vi "Binary.vi"(8 "Angle":dbl, 11 "General settings":T1) -> (2 "Binary":dbl[][](array[numeric]))   [LabVIEW 2014]
uses:
  Controls/SLM General Settings.ctl
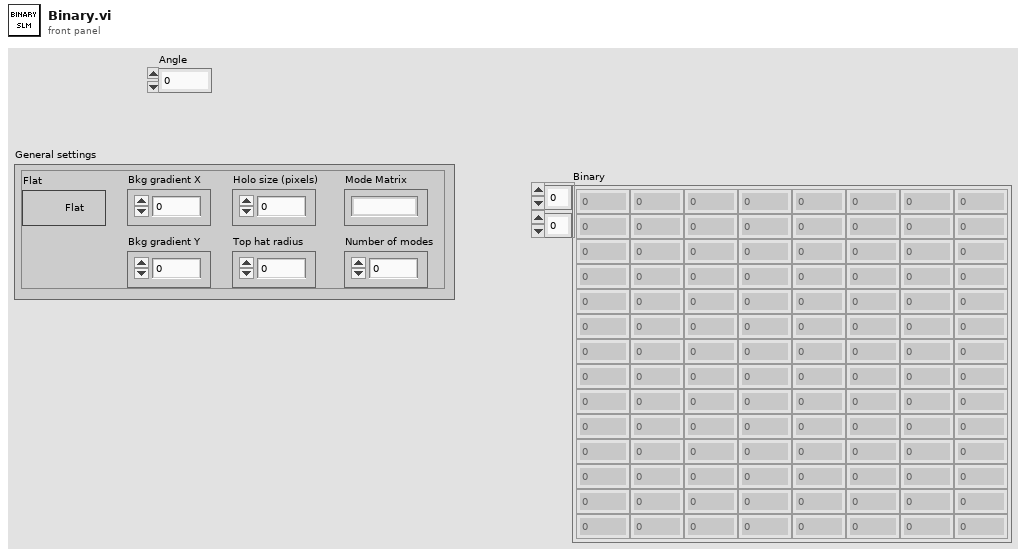
[diagram p1: front panel]
types:
  T1 = typedef "SLM General Settings.ctl" = cluster{"Holo size (pixels)":i32, "Top hat radius":dbl, "Number of modes":i32, "Bkg gradient X":dbl, "Bkg gradient Y":dbl, "Flat":bool, "Mode Matrix":u16}
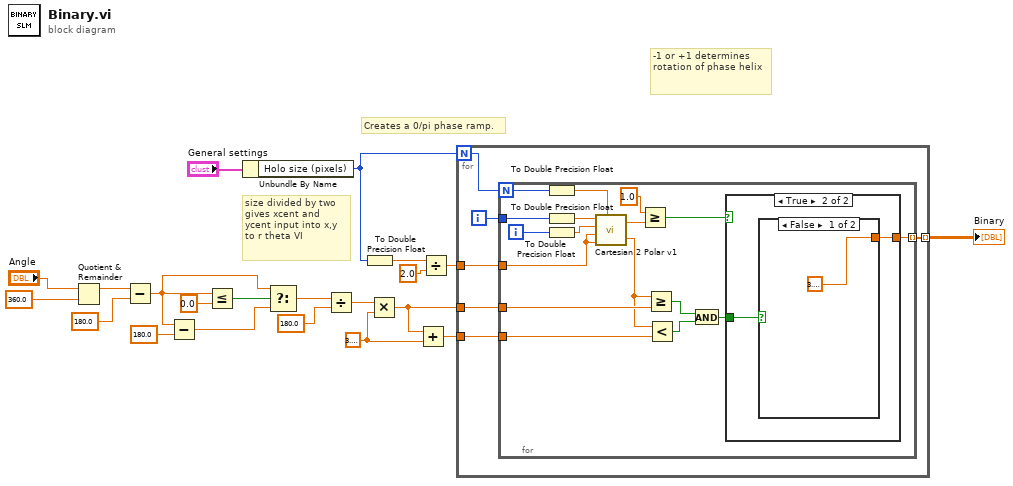
[diagram p0: block diagram]
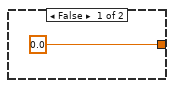
[diagram p2: hidden frame]
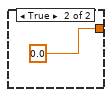
[diagram p3: hidden frame]
diagram:
  w4 = 3.141592653589793
  # "-1 or +1 determines \nrotation of phase helix"
  # "Creates a 0/pi phase ramp."
  # "size divided by two gives xcent and ycent input into x,y to r theta VI"
  n1 = Quotient & Remainder(x="Angle", y=360.0) -> (x-y*floor(x/y)=w12:dbl)  [unwired: 1 out]
  n2 = Subtract(x=w12, y=180.0) -> (x-y=w8:dbl)
  n3 = Subtract(x=w8, y=180.0) -> (x-y=w7:dbl)
  n4 = Less Or Equal?(x=w8, y=0.0) -> (x <= y?=w9:bool)
  n5 = Unbundle By Name("General settings") -> ("Holo size (pixels)"=w18:i32)
  n6 = Select(t=w8, s=w9, f=w7) -> (s? t:f=w6:dbl)
  n7 = Divide(x=w6, y=180.0) -> (x/y=w15:dbl)
  n8 = To Double Precision Float(number=w18) -> (double precision float=w17:dbl)
  n9 = Multiply(x=w15, y=w4) -> (x*y=w5:dbl)
  n10 = Add(x=w5, y=w4) -> (x+y=w3:dbl)
  n11 = Divide(x=w17, y=2.0) -> (x/y=w21:dbl)
  n12 = for {
    N: w18 -> [w24]
    tunnel: [w26] -> w1 mode=indexing
    tunnel: w21 -> [w25]
    tunnel: w5 -> [w23]
    tunnel: w3 -> [w22]
    i -> [w27]
    n13 = for {
      N: w24 -> [w38]
      tunnel: w27 -> [w43]
      tunnel: [w37] -> w26 mode=indexing
      tunnel: w25 -> [w39]
      tunnel: w23 -> [w33]
      tunnel: w22 -> [w32]
      i -> [w44]
      n14 = To Double Precision Float(number=w38) -> (double precision float=w36:dbl)
      n15 = To Double Precision Float(number=w43) -> (double precision float=w35:dbl)
      n16 = To Double Precision Float(number=w44) -> (double precision float=w34:dbl)
      n17 = call "Cartesian 2 Polar v1.vi"("x"=w35, "y"=w34, "xcent"=w39, "ycent"=w39, "diam"=w36) -> ("r"=w41:dbl, "t"=w28:dbl)
      n18 = Greater Or Equal?(x=1.0, y=w41) -> (x >= y?=w42:bool)
      n19 = Greater Or Equal?(x=w28, y=w33) -> (x >= y?=w30:bool)
      n20 = Less?(x=w28, y=w32) -> (x < y?=w31:bool)
      n21 = And(x=w30, y=w31) -> (x .and. y?=w29:bool)
      n22 = case shown="True" w42 {
        tunnel: [0.0 ("zernike") w46] -> w37
        tunnel: w29 -> [_ w47]
        frame False {
        }
        frame True {
          n23 = case shown="False" w47 {
            tunnel: [3.141592653589793 0.0] -> w46
            frame False {
            }
            frame True {
            }
          }
        }
      }
    }
  }
  "Binary" <- w1
